vi "Simple_Example_2Cam_IMAQ.vi"() -> ()   [LabVIEW 2019]
doc: "This example shows a simple recording of an image sequence and the image access afterwards for 2 cameras with identical resolution\nIt is a good starting point for writing multi camera applications.\nBut it will not be fail save, i.e. doesnt react on errors, just handles them forward to the end\n\nUsage:\nSelect your required image count before you start the program.\nOnce started, 2 camera classes will be initialized and images will be recorded automatically.\nWhen acquisition has finished you can address the images by index\nTo finish the program click on quit application, this will force fan exit of the camera class"
uses:
  camera/Camera.lvclass
panel:
  in  "Image Index 2":u32 max=9
  out "rawImage 2":u16[][](array[numeric])
  out "Recorded Images 2":u32
  out "Image 2":T1(plugin-control)
  out "rawImage":u16[][](array[numeric])
  out "Image":T1(plugin-control)
  in  "data_format":T2(ring)=enum."Mono16"
  in  "Image Index":u32 max=9
  out "Recorded Images":u32
  in  "Quit":bool
  out "Image Height":u16
  out "Image Width":u16
  in  "dwImgCount":u32=10 caption="Required Number of Images" max=4023
  out "Error":errorcluster {"code" format="%x"}
  # "This example shows a simple recording of an image sequence and the image access afterwards for 2 cameras with identical resolution\nIt is a good starting point for writing multi camera applications.\nBut it will not be fail save, i.e. doesnt react on errors, just handles them forward to the end\n\nUsage:\nSelect your required image count before you start the program.\nOnce started, 2 camera classes will be initialized and images will be recorded automatically.\nWhen acquisition has finished you can address the images by index\nTo finish the program click on quit application, this will force fan exit of the camera class"
  # "pco.labview"
  # "Camera Setup"
  # "Recording Control"
  # "Parameters for image readout"
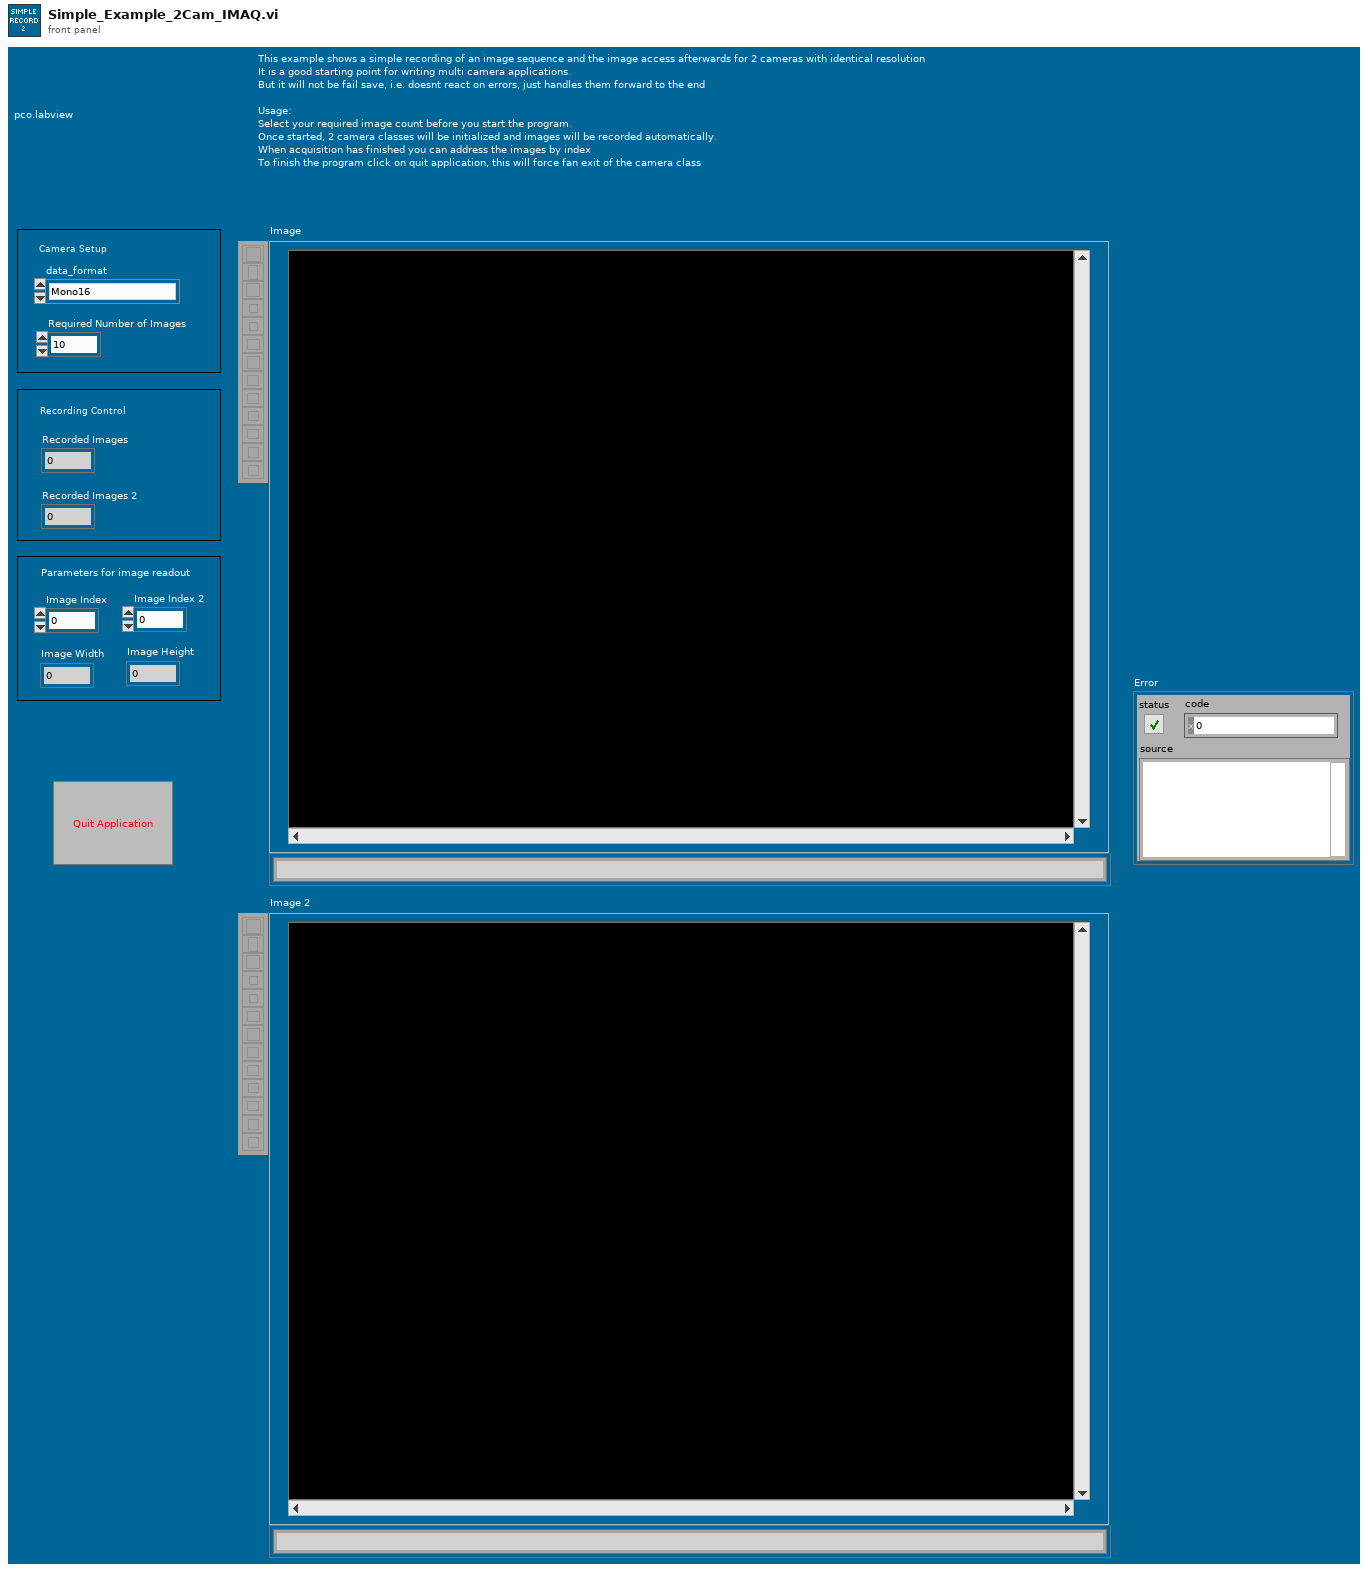
[diagram p1: front panel]
types:
  T1 = typedef "IMAQ Image.ctl" = refnum<image>
  T2 = enum16{"Undefined", "Mono8", "Mono16", "BGRA8", "RGBA8", "BGRA16", "RGBA16", "CompressedMono8"}
  T3 = enum8{"Enabled", "Disabled", "Disabled and Grayed Out"}
  T4 = cluster{"serial":u32, "type":u16, "sub_type":u16, "interface_type":u16, "bit_resolution":u16, "min_exposure_time_s":dbl, "max_exposure_time_s":dbl, "min_exposure_step_s":dbl, "min_delay_time_s":dbl, "max_delay_time_s":dbl, "min_delay_step_s":dbl, "min_width":u64, "min_height":u64, "max_width":u64, "max_height":u64, "roi_step_horz":u64, "roi_step_vert":u64, "roi_symmetric_horz":bool, "roi_symmetric_vert":bool, "has_timestamp_mode":bool, "has_timestamp_mode_ascii_only":bool, "pixelrate_vec":u32[], "conversion_factor_vec":sgl[], "has_trigger_mode_extexpctrl":bool, "has_acquire_mode":bool, "has_ext_acquire_mode":bool, "has_metadata_mode":bool, "has_ram":bool, "binning_horz_vec":u16[], "binning_vert_vec":u16[], "has_average_binning":bool, "pixel_format_vec":u32[]}
  T5 = typedef "Image Type" = u32
  T6 = typedef "Camera.lvclass/binning.ctl" = cluster{"vert":u16, "horz":u16, "mode":u16}
  T7 = cluster{"exposure_time_s":dbl, "delay_time_s":dbl, "roi":cluster{"x0":u64, "y0":u64, "x1":u64, "y1":u64}, "timestamp_mode":u16, "pixelrate":u32, "conversion_factor":sgl, "trigger_mode":u16, "acquire_mode":u16, "acquire_sequence_number":u32, "metadata_mode":u16, "noisefilter_mode":u16, "pixel_format":u32, "binning":T6, "auto_exposure":cluster{"region":u16, "min_exposure_s":dbl, "max_exposure_s":dbl}}
  T8 = enum16{"sequence", "sequence non blocking", "ring buffer", "fifo", "tif", "multitif", "pcoraw", "b16", "dicom", "multidicom", "camram_ring", "camram_segment"}
  T9 = cluster{"Plane 4 (alpha)":u16, "Plane 1 (Red)":u16, "Plane 2 (Green)":u16, "Plane 3 (Blue)":u16}[][]
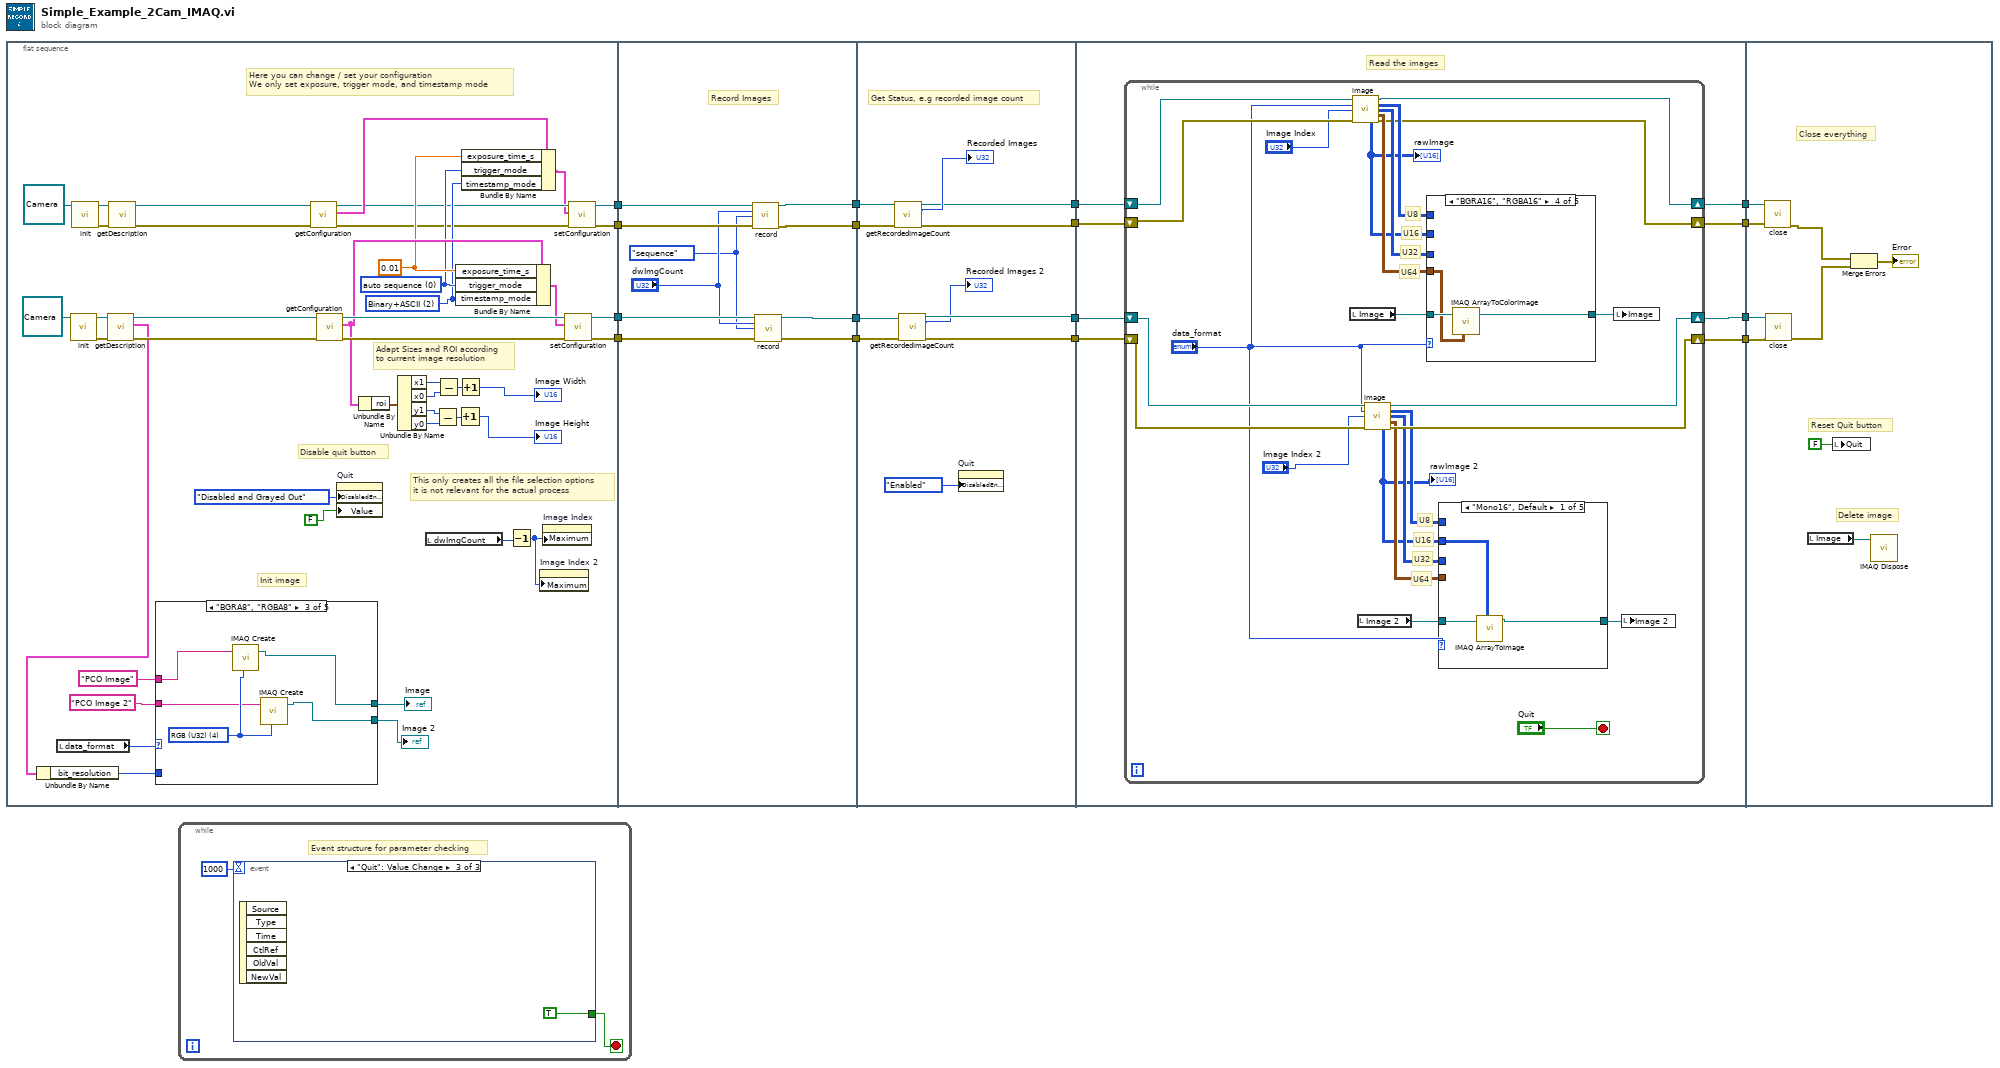
[diagram p0: block diagram]
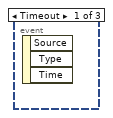
[diagram p2: hidden frame]
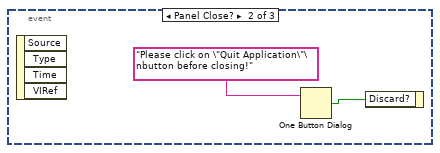
[diagram p3: hidden frame]
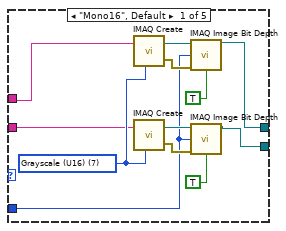
[diagram p4: hidden frame]
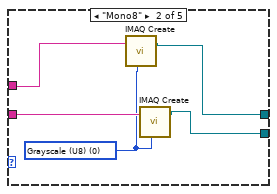
[diagram p5: hidden frame]
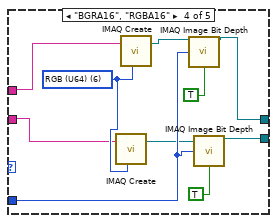
[diagram p6: hidden frame]
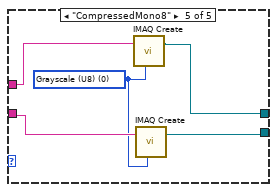
[diagram p7: hidden frame]
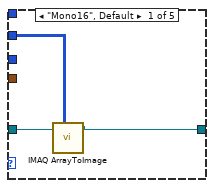
[diagram p8: hidden frame]
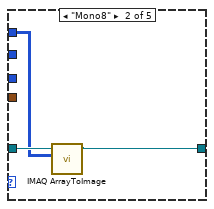
[diagram p9: hidden frame]
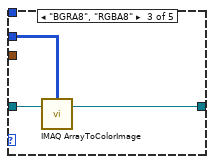
[diagram p10: hidden frame]
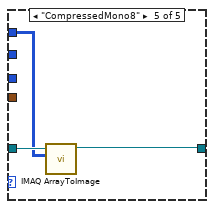
[diagram p11: hidden frame]
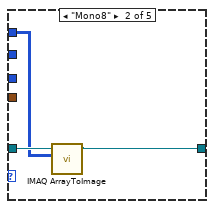
[diagram p12: hidden frame]
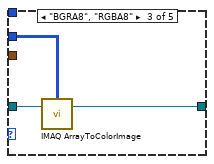
[diagram p13: hidden frame]
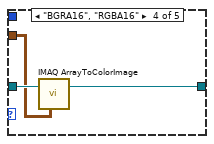
[diagram p14: hidden frame]
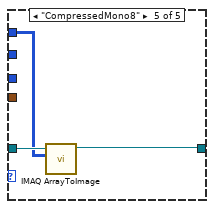
[diagram p15: hidden frame]
diagram:
  n1 = flat-sequence {
    tunnel: [w57] -> w16
    tunnel: [w56] -> w15
    tunnel: [w20] -> w8
    tunnel: [w19] -> w7
    tunnel: w16 -> [w108]
    tunnel: w15 -> [w107]
    tunnel: [w106] -> w14
    tunnel: [w105] -> w13
    tunnel: w8 -> [w104]
    tunnel: w7 -> [w103]
    tunnel: [w101] -> w6
    tunnel: [w100] -> w5
    tunnel: w14 -> [w119]
    tunnel: w13 -> [w118]
    tunnel: [w117] -> w12
    tunnel: [w116] -> w11
    tunnel: w6 -> [w113]
    tunnel: w5 -> [w112]
    tunnel: [w110] -> w4
    tunnel: [w109] -> w3
    tunnel: w12 -> [w126]
    tunnel: w11 -> [w127]
    tunnel: [w125] -> w10
    tunnel: [w124] -> w9
    tunnel: w4 -> [w123]
    tunnel: w3 -> [w122]
    tunnel: [w121] -> w2
    tunnel: [w120] -> w1
    tunnel: w10 -> [w189]
    tunnel: w9 -> [w188]
    tunnel: w2 -> [w186]
    tunnel: w1 -> [w185]
    frame #0 {
      w26 = 0.01 ("exposure_time_s")
      w24 = u16 2 items=["OFF", "Binary", "Binary+ASCII", "ASCII"] ("TimestampMode")
      w25 = u16 0 items=["auto sequence"=0, "software trigger"=1, "external exposure start & software trigger"=2, "external exposure control"=3, "external synchronized"=4, "fast external exposure control"=5, "external CDS control"=6, "slow external exposure control"=7, "external synchronized HDSDI"=258] ("TriggerMode")
      # "Here you can change / set your configuration\nWe only set exposure, trigger mode, and timestamp mode"
      # "Init image"
      # "This only creates all the file selection options\nit is not relevant for the actual process"
      # "Adapt Sizes and ROI according\nto current image resolution"
      # "Disable quit button"
      n2 = local read "data_format"() -> (w42:T2)
      n3 = call-dynamic "init.vi"("Camera in"=refnum<class "Camera.lvclass"> refnum ("PCOCamera in")) -> ("Camera out"=w38:refnum<class "Camera.lvclass">, "error out"=w39:errorcluster)  [unwired: 8 in]
      n4 = call-dynamic "init.vi"("Camera in"=refnum<class "Camera.lvclass"> refnum ("PCOCamera in")) -> ("Camera out"=w30:refnum<class "Camera.lvclass">, "error out"=w31:errorcluster)  [unwired: 8 in]
      n5 = call-dynamic "getDescription.vi"("error in (no error)"=w39, "Camera in"=w38) -> ("error out"=w36:errorcluster, "description"=w35:T4, "Camera out"=w37:refnum<class "Camera.lvclass">)  [unwired: 7 in]
      n6 = Unbundle By Name(w35) -> ("bit_resolution"=w34:u16)
      n7 = call-dynamic "getDescription.vi"("error in (no error)"=w31, "Camera in"=w30) -> ("error out"=w28:errorcluster, "Camera out"=w29:refnum<class "Camera.lvclass">)  [unwired: 7 in, 1 out]
      n8 = case shown="\"BGRA8\", \"RGBA8\"" w42 {
        tunnel: "PCO Image 2" ("Image Name") -> [w65 w78 w82 w87 w98]
        tunnel: [w64 w75 w80 w85 w95] -> w41
        tunnel: w34 -> [w67 _ _ w90 _]
        tunnel: [w63 w76 w81 w86 w96] -> w33
        tunnel: "PCO Image" ("Image Name") -> [w62 w74 w79 w84 w94]
        frame "Mono16", Default {
          w66 = T5 7 items=["Grayscale (U8)", "Grayscale (I16)", "Grayscale (SGL)", "Complex (CSG)", "RGB (U32)", "HSL (U32)", "RGB (U64)", "Grayscale (U16)"] ("Image Type")
          n9 = call "IMAQ Create"("Image Name"=w62, "Image Type"=w66) -> ("New Image"=w69:T1, "error out"=w70:errorcluster)  [unwired: 3 in]
          n10 = call "IMAQ Create"("Image Name"=w65, "Image Type"=w66) -> ("New Image"=w72:T1, "error out"=w71:errorcluster)  [unwired: 3 in]
          n11 = call "IMAQ Image Bit Depth"("Image"=w69, "Bit Depth (0)"=w67, "error in (no error)"=w70, "Get/Set Bit Depth? (Set)"=TRUE) -> ("Image Out"=w64:T1)  [unwired: 9 in, 2 out]
          n12 = call "IMAQ Image Bit Depth"("Image"=w72, "Bit Depth (0)"=w67, "error in (no error)"=w71, "Get/Set Bit Depth? (Set)"=TRUE) -> ("Image Out"=w63:T1)  [unwired: 9 in, 2 out]
        }
        frame "Mono8" {
          w77 = T5 0 items=["Grayscale (U8)", "Grayscale (I16)", "Grayscale (SGL)", "Complex (CSG)", "RGB (U32)", "HSL (U32)", "RGB (U64)", "Grayscale (U16)"] ("Image Type")
          n13 = call "IMAQ Create"("Image Name"=w74, "Image Type"=w77) -> ("New Image"=w75:T1)  [unwired: 3 in, 1 out]
          n14 = call "IMAQ Create"("Image Name"=w78, "Image Type"=w77) -> ("New Image"=w76:T1)  [unwired: 3 in, 1 out]
        }
        frame "BGRA8", "RGBA8" {
          w83 = T5 4 items=["Grayscale (U8)", "Grayscale (I16)", "Grayscale (SGL)", "Complex (CSG)", "RGB (U32)", "HSL (U32)", "RGB (U64)", "Grayscale (U16)"] ("Image Type")
          n15 = call "IMAQ Create"("Image Name"=w79, "Image Type"=w83) -> ("New Image"=w80:T1)  [unwired: 3 in, 1 out]
          n16 = call "IMAQ Create"("Image Name"=w82, "Image Type"=w83) -> ("New Image"=w81:T1)  [unwired: 3 in, 1 out]
        }
        frame "BGRA16", "RGBA16" {
          w88 = T5 6 items=["Grayscale (U8)", "Grayscale (I16)", "Grayscale (SGL)", "Complex (CSG)", "RGB (U32)", "HSL (U32)", "RGB (U64)", "Grayscale (U16)"] ("Image Type")
          n17 = call "IMAQ Create"("Image Name"=w87, "Image Type"=w88) -> ("New Image"=w89:T1)  [unwired: 3 in, 1 out]
          n18 = call "IMAQ Create"("Image Name"=w84, "Image Type"=w88) -> ("New Image"=w92:T1)  [unwired: 3 in, 1 out]
          n19 = call "IMAQ Image Bit Depth"("Image"=w92, "Bit Depth (0)"=w90, "Get/Set Bit Depth? (Set)"=TRUE) -> ("Image Out"=w85:T1)  [unwired: 10 in, 2 out]
          n20 = call "IMAQ Image Bit Depth"("Image"=w89, "Bit Depth (0)"=w90, "Get/Set Bit Depth? (Set)"=TRUE) -> ("Image Out"=w86:T1)  [unwired: 10 in, 2 out]
        }
        frame "CompressedMono8" {
          w97 = T5 0 items=["Grayscale (U8)", "Grayscale (I16)", "Grayscale (SGL)", "Complex (CSG)", "RGB (U32)", "HSL (U32)", "RGB (U64)", "Grayscale (U16)"] ("Image Type")
          n21 = call "IMAQ Create"("Image Name"=w94, "Image Type"=w97) -> ("New Image"=w95:T1)  [unwired: 3 in, 1 out]
          n22 = call "IMAQ Create"("Image Name"=w98, "Image Type"=w97) -> ("New Image"=w96:T1)  [unwired: 3 in, 1 out]
        }
      }
      "Image" <- w41
      "Image 2" <- w33
      n23 = call-dynamic "getConfiguration.vi"("error in (no error)"=w28, "Camera in"=w29) -> ("error out"=w22:errorcluster, "configuration"=w27:T7, "Camera out"=w23:refnum<class "Camera.lvclass">)  [unwired: 7 in]
      n24 = call-dynamic "getConfiguration.vi"("error in (no error)"=w36, "Camera in"=w37) -> ("error out"=w59:errorcluster, "configuration"=w55:T7, "Camera out"=w60:refnum<class "Camera.lvclass">)  [unwired: 7 in]
      n25 = property on="Quit" class="Bool (strict)"("DisabledEnum"=T3."Disabled and Grayed Out" ("Disabled"), "Value"=FALSE ("Stop")) -> ()  [unwired: 2 in, 2 out]
      n26 = Unbundle By Name(w55) -> ("roi"=w54:cluster{"x0":u64, "y0":u64, "x1":u64, "y1":u64})
      n27 = Unbundle By Name(w54) -> ("x1"=w52:u64, "x0"=w53:u64, "y1"=w50:u64, "y0"=w51:u64)
      n28 = local read "dwImgCount"() -> (w43:u32)
      n29 = Subtract(x=w50, y=w51) -> (x-y=w48:u64)
      n30 = Subtract(x=w52, y=w53) -> (x-y=w49:u64)
      n31 = Bundle By Name(cluster=w55, "exposure_time_s"=w26, "trigger_mode"=w25, "timestamp_mode"=w24) -> (w58:T7)
      n32 = Increment(x=w48) -> (x+1=→"Image Height":u64)
      n33 = Increment(x=w49) -> (x+1=→"Image Width":u64)
      n34 = Bundle By Name(cluster=w27, "exposure_time_s"=w26, "trigger_mode"=w25, "timestamp_mode"=w24) -> (w21:T7)
      n35 = Decrement(x=w43) -> (x-1=w17:u32)
      n36 = property on="Image Index 2" class="DigNum (strict)"("Maximum"=w17) -> ()  [unwired: 2 in, 2 out]
      n37 = property on="Image Index" class="DigNum (strict)"("Maximum"=w17) -> ()  [unwired: 2 in, 2 out]
      n38 = call-dynamic "setConfiguration.vi"("error in (no error)"=w59, "configuration"=w58, "Camera in"=w60) -> ("error out"=w56:errorcluster, "Camera out"=w57:refnum<class "Camera.lvclass">)  [unwired: 7 in]
      n39 = call-dynamic "setConfiguration.vi"("error in (no error)"=w22, "configuration"=w21, "Camera in"=w23) -> ("error out"=w19:errorcluster, "Camera out"=w20:refnum<class "Camera.lvclass">)  [unwired: 7 in]
    }
    frame #1 {
      w99 = T8."sequence" ("record_mode")
      # "Record Images"
      n40 = call-dynamic "record.vi"("Camera in"=w104, "num_images"="dwImgCount", "record_mode"=w99, "error in (no error)"=w103) -> ("Camera out"=w101:refnum<class "Camera.lvclass">, "error out"=w100:errorcluster)  [unwired: 10 in]
      n41 = call-dynamic "record.vi"("Camera in"=w108, "num_images"="dwImgCount", "record_mode"=w99, "error in (no error)"=w107) -> ("Camera out"=w106:refnum<class "Camera.lvclass">, "error out"=w105:errorcluster)  [unwired: 10 in]
    }
    frame #2 {
      # "Get Status, e.g recorded image count"
      n42 = call-dynamic "getRecordedImageCount.vi"("Camera in"=w113, "error in (no error)"=w112) -> ("Camera out"=w110:refnum<class "Camera.lvclass">, "recorded_image_count"=→"Recorded Images":u32, "error out"=w109:errorcluster)  [unwired: 11 in]
      n43 = call-dynamic "getRecordedImageCount.vi"("Camera in"=w119, "error in (no error)"=w118) -> ("Camera out"=w117:refnum<class "Camera.lvclass">, "recorded_image_count"=→"Recorded Images 2":u32, "error out"=w116:errorcluster)  [unwired: 11 in]
      n44 = property on="Quit" class="Bool (strict)"("DisabledEnum"=T3."Enabled" ("Disabled")) -> ()  [unwired: 2 in, 2 out]
    }
    frame #3 {
      # "Read the images"
      n45 = while {
        shift-right: [w149] -> w125
        shift-left: w126 -> [w151]
        shift-right: [w148] -> w124
        shift-left: w127 -> [w150]
        shift-right: [w131] -> w121
        shift-left: w123 -> [w134]
        shift-right: [w132] -> w120
        shift-left: w122 -> [w133]
        stop <- "Quit" stop-if-true
        # "U64"
        # "U32"
        # "U16"
        # "U8"
        # "U64"
        # "U32"
        # "U16"
        # "U8"
        n46 = local read "Image"() -> (w140:T1)
        n47 = call-dynamic "image.vi"("Camera in"=w134, "data_format"="data_format", "image_index"="Image Index", "error in (no error)"=w133) -> ("Camera out"=w131:refnum<class "Camera.lvclass">, "image (U8)"=w137:u8[][], "image (U32)"=w138:u32[][], "image (U64)"=w139:T9, "raw_image (U16)"=w135:u16[][], "error out"=w132:errorcluster)  [unwired: 3 in, 3 out]
        "rawImage" <- w135
        n48 = local read "Image 2"() -> (w144:T1)
        n49 = call-dynamic "image.vi"("Camera in"=w151, "data_format"="data_format", "image_index"="Image Index 2", "error in (no error)"=w150) -> ("Camera out"=w149:refnum<class "Camera.lvclass">, "image (U8)"=w147:u8[][], "image (U32)"=w146:u32[][], "image (U64)"=w145:T9, "raw_image (U16)"=w136:u16[][], "error out"=w148:errorcluster)  [unwired: 3 in, 3 out]
        "rawImage 2" <- w136
        n50 = case shown="\"BGRA16\", \"RGBA16\"" "data_format" {
          tunnel: w140 -> [w154 w157 w160 w163 w166]
          tunnel: [w152 w155 w159 w161 w165] -> w141
          tunnel: w139 -> [_ _ _ w162 _]
          tunnel: w138 -> [_ _ w158 _ _]
          tunnel: w137 -> [_ w156 _ _ w164]
          tunnel: w135 -> [w153 _ _ _ _]
          frame "Mono16", Default {
            n51 = call "IMAQ ArrayToImage"("Image Pixels (U16)"=w153, "Image"=w154) -> ("Image Out"=w152:T1)  [unwired: 8 in, 1 out]
          }
          frame "Mono8" {
            n52 = call "IMAQ ArrayToImage"("Image Pixels (U8)"=w156, "Image"=w157) -> ("Image Out"=w155:T1)  [unwired: 8 in, 1 out]
          }
          frame "BGRA8", "RGBA8" {
            n53 = call "IMAQ ArrayToColorImage"("Image Pixels (U32)"=w158, "Image"=w160) -> ("Image Out"=w159:T1)  [unwired: 3 in, 1 out]
          }
          frame "BGRA16", "RGBA16" {
            n54 = call "IMAQ ArrayToColorImage"("Image"=w163, "Image Pixels (U64)"=w162) -> ("Image Out"=w161:T1)  [unwired: 3 in, 1 out]
          }
          frame "CompressedMono8" {
            n55 = call "IMAQ ArrayToImage"("Image Pixels (U8)"=w164, "Image"=w166) -> ("Image Out"=w165:T1)  [unwired: 8 in, 1 out]
          }
        }
        n56 = case shown="\"Mono16\", Default" "data_format" {
          tunnel: w144 -> [w169 w172 w175 w178 w181]
          tunnel: [w167 w170 w174 w176 w180] -> w143
          tunnel: w145 -> [_ _ _ w177 _]
          tunnel: w146 -> [_ _ w173 _ _]
          tunnel: w147 -> [_ w171 _ _ w179]
          tunnel: w136 -> [w168 _ _ _ _]
          frame "Mono16", Default {
            n57 = call "IMAQ ArrayToImage"("Image Pixels (U16)"=w168, "Image"=w169) -> ("Image Out"=w167:T1)  [unwired: 8 in, 1 out]
          }
          frame "Mono8" {
            n58 = call "IMAQ ArrayToImage"("Image Pixels (U8)"=w171, "Image"=w172) -> ("Image Out"=w170:T1)  [unwired: 8 in, 1 out]
          }
          frame "BGRA8", "RGBA8" {
            n59 = call "IMAQ ArrayToColorImage"("Image Pixels (U32)"=w173, "Image"=w175) -> ("Image Out"=w174:T1)  [unwired: 3 in, 1 out]
          }
          frame "BGRA16", "RGBA16" {
            n60 = call "IMAQ ArrayToColorImage"("Image"=w178, "Image Pixels (U64)"=w177) -> ("Image Out"=w176:T1)  [unwired: 3 in, 1 out]
          }
          frame "CompressedMono8" {
            n61 = call "IMAQ ArrayToImage"("Image Pixels (U8)"=w179, "Image"=w181) -> ("Image Out"=w180:T1)  [unwired: 8 in, 1 out]
          }
        }
        n62 = local write "Image"(w141) -> ()
        n63 = local write "Image 2"(w143) -> ()
      }
    }
    frame #4 {
      # "Delete image"
      # "Reset Quit button"
      # "Close everything"
      n64 = call-dynamic "close.vi"("error in (no error)"=w185, "Camera in"=w186) -> ("error out"=w183:errorcluster)  [unwired: 9 in]
      n65 = call-dynamic "close.vi"("error in (no error)"=w188, "Camera in"=w189) -> ("error out"=w182:errorcluster)  [unwired: 9 in]
      n66 = local read "Image"() -> (w187:T1)
      n67 = local write "Quit"(FALSE ("Stop")) -> ()
      n68 = Merge Errors(w183, w182) -> (→"Error":errorcluster)
      n69 = call "IMAQ Dispose"("Image"=w187) -> ()  [unwired: 5 in, 1 out]
    }
  }
  n70 = while {
    stop <- w191 stop-if-true
    # "Event structure for parameter checking"
    n71 = event shown="[2] \"Quit\": Value Change" {
      selector: _ -> [_ _ _]
      dyn-events: _ -> [_ _ _]
      timeout: 1000 -> [_ _ _]
      tunnel: [_ _ TRUE] -> w191
      event Timeout {
        n72 = event-data() -> ()  [unwired: 1 in, 3 out]
      }
      event Panel Close? {
        n73 = event-data() -> ()  [unwired: 1 in, 4 out]
        n74 = One Button Dialog(message="Please click on \"Quit Application\"\nbutton before closing!") -> (true=w193:bool)  [unwired: 1 in]
        n75 = event-data("Discard?"=w193) -> ()  [unwired: 1 in, 1 out]
      }
      event "Quit": Value Change {
        n76 = event-data() -> ()  [unwired: 1 in, 6 out]
      }
    }
  }
